vi "test File Save Load.vi"(8 "error in (no error)":errorcluster, 11 "TestCase in":refnum<class "Configuration Tests.lvclass">) -> (0 "error out":errorcluster, 3 "TestCase out":refnum<class "Configuration Tests.lvclass">)   [LabVIEW 2019, in "Configuration Tests.lvclass"]
uses:
  Configuration Tests.lvclass
  Configuration Tests.lvclass/Configuration Tests.ctl
  Classes/Configuration Session/Configuration Session.lvclass
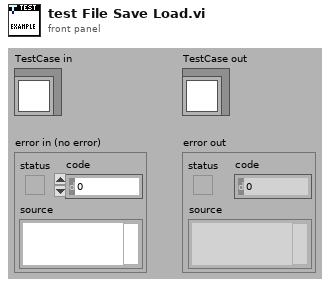
[diagram p1: front panel]
types:
  T1 = typedef "DSF Core.lvlib/DSF Engine Framework Configuration.ctl" = cluster{"plugins":T2[]}
  T2 = typedef "DSF Core.lvlib/DSF Engine Plugin Configuration.ctl" = cluster{"core":T3, "component settings":T5[], "threads":T6[]}
  T3 = typedef "DSF Core.lvlib/Plugin Configuration.lvclass/Core Plugin Configuration.ctl" = cluster{"name":string, "components":string[], "cycle timing":T4}
  T4 = typedef "DSF Core.lvlib/DSF Timing Info.ctl" = cluster{"priority":u64, "decimation":u64, "offset":u64}
  T5 = typedef "DSF Core.lvlib/DSF Settings Info.ctl" = cluster{"component":string, "values":cluster{"key":string, "value":string}[]}
  T6 = typedef "DSF Core.lvlib/DSF Engine Plugin Thread Configuration.ctl" = cluster{"core":T7, "component settings":T5[], "transfer groups":T8[]}
  T7 = typedef "DSF Core.lvlib/Thread Configuration.lvclass/Core Thread Configuration.ctl" = cluster{"processor":i32, "priority offset":i16}
  T8 = typedef "DSF Core.lvlib/DSF Engine Transfer Group Configuration.ctl" = cluster{"core":T9, "component settings":T5[], "transfers":T12[]}
  T9 = typedef "DSF Core.lvlib/Group Configuration.lvclass/Core Group Configuration.ctl" = cluster{"name":string, "direction":T10, "cycle timing":T4, "timeout behavior":T11, "enable conversion":bool}
  T10 = typedef "DSF Core.lvlib/DSF Direction.ctl" = enum8{"Tx", "Rx"}
  T11 = typedef "DSF Core.lvlib/DSF Timeout Behavior.ctl" = enum8{"Increment Late Count", "Throw Error"}
  T12 = typedef "DSF Core.lvlib/DSF Engine Transfer Configuration.ctl" = cluster{"core":T13, "component settings":T5[], "channels":T14[]}
  T13 = typedef "DSF Core.lvlib/Transfer Configuration.lvclass/Core Transfer Configuration.ctl" = cluster{"name":string}
  T14 = typedef "DSF Core.lvlib/DSF Engine Channel Configuration.ctl" = cluster{"core":T15, "component settings":T5[]}
  T15 = typedef "DSF Core.lvlib/Channel Configuration.lvclass/Core Channel Configuration.ctl" = cluster{"name":string, "units":string, "engine data type":T16, "string data type":T16, "string offset":u64}
  T16 = typedef "DSF Core.lvlib/DSF Data Type.ctl" = enum8{"Bool", "SGL", "DBL", "I8", "I16", "I32", "I64", "U8", "U16", "U32", "U64"}
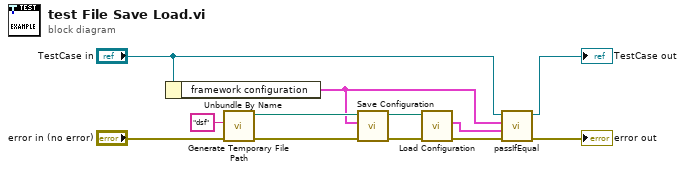
[diagram p0: block diagram]
diagram:
  n1 = Unbundle By Name("TestCase in") -> ("framework configuration"=w2:T1)
  n2 = call <vilib>:"Generate Temporary File Path.vi"("error in (no error)"="error in (no error)", "Temporary File Extension (tmp)"="dsf") -> ("error out"=w5:errorcluster, "Unique Temporary File Path"=w4:path)  [unwired: 8 in]
  n3 = call "Save Configuration.vi"("error in (no error)"=w5, "framework configuration"=w2, "configuration file path"=w4) -> ("error out"=w9:errorcluster, "configuration file path dup"=w10:path)  [unwired: 5 in, 2 out]
  n4 = call "Load Configuration.vi"("error in (no error)"=w9, "configuration file path"=w10) -> ("error out"=w8:errorcluster, "framework configuration"=w1:T1)  [unwired: 6 in, 2 out]
  n5 = call-dynamic "passIfEqual.vi"("error in (no error)"=w8, "y"=w1, "x"=w2, "TestCase in"="TestCase in") -> ("error out"=→"error out":errorcluster, "TestCase out"=→"TestCase out":refnum<class "Configuration Tests.lvclass">)  [unwired: 6 in]
